vi "Set Crop ROI.vi"(8 "error in (no error)":errorcluster, 11 "Frame Grabber Data in":T2={"Camera Session"="", "Frame"=refnum, "AVI Refnum"=refnum, "Codecs"=[], "Frame number"=0, "Tracking File Refnum"=refnum, "Tick Count"=0, "Probe Object"=refnum, "Playback Probe Data"=[], "Rigid Body"={"Position"={"x (mm)"=0.0, "y (mm)"=0.0, "z (mm)"=0.0}, "Orientation"={"Pitch (rad)"=0.0, "Yaw (rad)"=0.0, "Roll (rad)"=0.0}, "Quaternion"={"qx"=0.0, "qy"=0.0, "qz"=0.0, "qw"=0.0}, "Tracked?"=FALSE}, "Total no frames playback"=0, "Video FPS"=0.0, "Camera connected?"=FALSE, "Scene"=refnum, "Cropped Frame"=refnum, "Tracker FPS"=0.0, "Crop ROI"=[], "Presentation Values"=[], "Elapsed time (ms)"=0, "Camera frames playback"=0, "Refnums"={"Live Refnum"=refnum, "Record Refnum"=refnum, "Recording Settings Refnum"=refnum, "Playback Refnum"=refnum, "Frame Slider Refnum"=refnum, "Pause Refnum"=refnum, "Home Refnum"=refnum, "Crop Refnum"=refnum, "Clear Crop Refnum"=refnum, "stop refnum"=refnum, "Playback Rate Refnum"=refnum, "Operator Settings Refnums"=refnum, "Presentation Refnum"=refnum, "Gestation Refnum"=refnum, "Connection Settings Refnum"=refnum, "Crop Time Frame Slider Refnum"=refnum, "Cancel Save Refnum"=refnum}, "Dimensions"={"Probe Dimensions"={"Probe Width"=0.0, "Probe Depth"=1.0, "Probe Height"=0.0}, "Room Dimensions"={"Room Width"=0.0, "Room Depth"=0.0, "Room Height"=0.0}}, "Playback Data As Strings"=[], "Cropped Tracking File Refnum"=refnum, "Cropped AVI Refnum"=refnum, "Header"=[]}) -> (0 "error out":errorcluster, 1 "Crop ROI":i32[](array[numeric]), 2 "Image Out":T1, 3 "Frame Grabber Data out":T2={"Camera Session"="", "Frame"=refnum, "AVI Refnum"=refnum, "Codecs"=[], "Frame number"=0, "Tracking File Refnum"=refnum, "Tick Count"=0, "Probe Object"=refnum, "Playback Probe Data"=[], "Rigid Body"={"Position"={"x (mm)"=0.0, "y (mm)"=0.0, "z (mm)"=0.0}, "Orientation"={"Pitch (rad)"=0.0, "Yaw (rad)"=0.0, "Roll (rad)"=0.0}, "Quaternion"={"qx"=0.0, "qy"=0.0, "qz"=0.0, "qw"=0.0}, "Tracked?"=FALSE}, "Total no frames playback"=0, "Video FPS"=0.0, "Camera connected?"=FALSE, "Scene"=refnum, "Cropped Frame"=refnum, "Tracker FPS"=0.0, "Crop ROI"=[], "Presentation Values"=[], "Elapsed time (ms)"=0, "Camera frames playback"=0, "Refnums"={"Live Refnum"=refnum, "Record Refnum"=refnum, "Recording Settings Refnum"=refnum, "Playback Refnum"=refnum, "Frame Slider Refnum"=refnum, "Pause Refnum"=refnum, "Home Refnum"=refnum, "Crop Refnum"=refnum, "Clear Crop Refnum"=refnum, "stop refnum"=refnum, "Playback Rate Refnum"=refnum, "Operator Settings Refnums"=refnum, "Presentation Refnum"=refnum, "Gestation Refnum"=refnum, "Connection Settings Refnum"=refnum, "Crop Time Frame Slider Refnum"=refnum, "Cancel Save Refnum"=refnum}, "Dimensions"={"Probe Dimensions"={"Probe Width"=0.0, "Probe Depth"=1.0, "Probe Height"=0.0}, "Room Dimensions"={"Room Width"=0.0, "Room Depth"=0.0, "Room Height"=0.0}}, "Playback Data As Strings"=[], "Cropped Tracking File Refnum"=refnum, "Cropped AVI Refnum"=refnum, "Header"=[]}, 5 "Zero crop size?":bool)   [LabVIEW 2017]
uses:
  Controls/Frame Grabber Data.ctl
  <vilib>/userdefined/High Color/IMAQdx.ctl
  <vilib>/vision/Image Controls.llb/IMAQ Image.ctl
  <vilib>/vision/Avi.llb/IMAQ AVI2 Refnum.ctl
  Controls/Rigid Body Info.ctl
  Controls/Position.ctl
  Controls/Orientation.ctl
  Controls/Refnums.ctl
  Controls/Recording Settings.ctl
  Controls/Operator Settings.ctl
  Controls/Operator.ctl
  Controls/Dimensions.ctl
  Controls/Room Dimensions.ctl
  <vilib>/vision/NI_Vision_Development_Module.lvlib
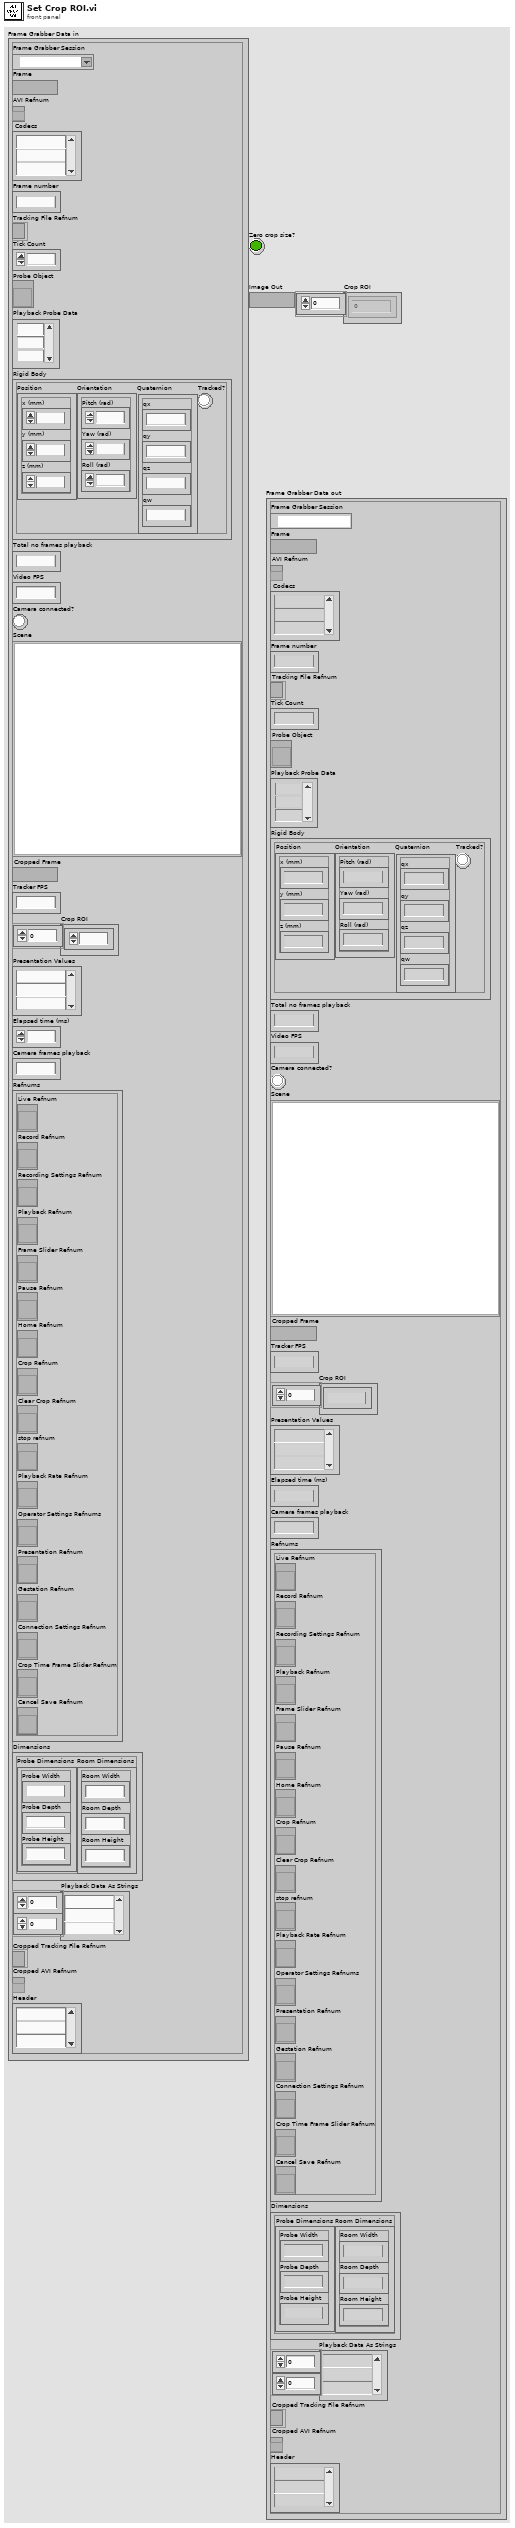
[diagram p1: front panel]
types:
  T1 = typedef "IMAQ Image.ctl" = refnum<image>
  T2 = typedef "Frame Grabber Data.ctl" = cluster{"Camera Session":T3, "Frame":T1, "AVI Refnum":T4, "Codecs":string[], "Frame number":u32, "Tracking File Refnum":refnum<file>, "Tick Count":u32, "Probe Object":refnum<vi>, "Playback Probe Data":dbl[][], "Rigid Body":T5, "Total no frames playback":i32, "Video FPS":dbl, "Camera connected?":bool, "Scene":refnum<vi>, "Cropped Frame":T1, "Tracker FPS":dbl, "Crop ROI":i32[], "Presentation Values":string[], "Elapsed time (ms)":u32, "Camera frames playback":u32, "Refnums":T8, "Dimensions":T9, "Playback Data As Strings":string[][], "Cropped Tracking File Refnum":refnum<file>, "Cropped AVI Refnum":T4, "Header":string[]}
  T3 = typedef "IMAQdx.ctl" = refnum<k21>
  T4 = typedef "IMAQ AVI2 Refnum.ctl" = refnum<k20>
  T5 = typedef "Rigid Body Info.ctl" = cluster{"Position":T6, "Orientation":T7, "Quaternion":cluster{"qx":sgl, "qy":sgl, "qz":sgl, "qw":sgl}, "Tracked?":bool}
  T6 = typedef "Position.ctl" = cluster{"x (mm)":sgl, "y (mm)":sgl, "z (mm)":sgl}
  T7 = typedef "Orientation.ctl" = cluster{"Pitch (rad)":sgl, "Yaw (rad)":sgl, "Roll (rad)":sgl}
  T8 = typedef "Refnums.ctl" = cluster{"Live Refnum":refnum<vi>, "Record Refnum":refnum<vi>, "Recording Settings Refnum":refnum<vi>, "Playback Refnum":refnum<vi>, "Frame Slider Refnum":refnum<vi>, "Pause Refnum":refnum<vi>, "Home Refnum":refnum<vi>, "Crop Refnum":refnum<vi>, "Clear Crop Refnum":refnum<vi>, "stop refnum":refnum<vi>, "Playback Rate Refnum":refnum<vi>, "Operator Settings Refnums":refnum<vi>, "Presentation Refnum":refnum<vi>, "Gestation Refnum":refnum<vi>, "Connection Settings Refnum":refnum<vi>, "Crop Time Frame Slider Refnum":refnum<vi>, "Cancel Save Refnum":refnum<vi>}
  T9 = typedef "Dimensions.ctl" = cluster{"Probe Dimensions":cluster{"Probe Width":sgl, "Probe Depth":sgl, "Probe Height":sgl}, "Room Dimensions":T10}
  T10 = typedef "Room Dimensions.ctl" = cluster{"Room Width":dbl, "Room Depth":dbl, "Room Height":dbl}
  T11 = typedef "IMAQ Rectangle" = cluster{"Left":i32, "Top":i32, "Right":i32, "Bottom":i32, "Rotation":dbl}
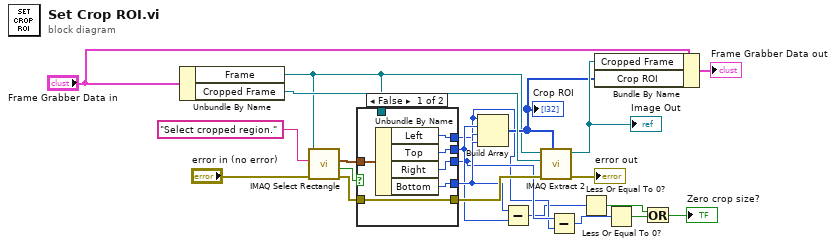
[diagram p0: block diagram]
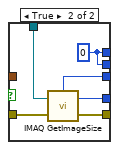
[diagram p2: hidden frame]
diagram:
  n1 = Unbundle By Name("Frame Grabber Data in") -> ("Frame"=w10:T1, "Cropped Frame"=w17:T1)
  n2 = call "IMAQ Select Rectangle"("error in (no error)"="error in (no error)", "Prompt"="Select cropped region.", "Image In"=w10) -> ("error out"=w12:errorcluster, "Cancelled"=w13:bool, "Rectangle"=w22:T11)  [unwired: 5 in, 1 out]
  n3 = case shown="False" w13 {
    tunnel: w22 -> [w28 _]
    tunnel: [w27 w32] -> w6
    tunnel: [w26 w32] -> w8
    tunnel: [w25 w30] -> w7
    tunnel: [w24 w31] -> w9
    tunnel: w12 -> [w23 w34]
    tunnel: [w23 w33] -> w11
    tunnel: w10 -> [_ w29]
    frame False {
      n4 = Unbundle By Name(w28) -> ("Left"=w27:i32, "Top"=w26:i32, "Right"=w25:i32, "Bottom"=w24:i32)
    }
    frame True {
      w32 = 0 ("Left")
      n5 = call "IMAQ GetImageSize"("Image"=w29, "error in (no error)"=w34) -> ("Y Resolution"=w31:i32, "X Resolution"=w30:i32, "error out"=w33:errorcluster)  [unwired: 2 in]
    }
  }
  n6 = Build Array(w6, w8, w7, w9) -> (w14:i32[])
  "Crop ROI" <- w14
  n7 = Subtract(x=w9, y=w8) -> (x-y=w4:i32)
  n8 = call "IMAQ Extract 2"("Optional Rectangle"=w14, "error in (no error)"=w11, "Image Dst"=w17, "Image Src"=w10) -> ("error out"=→"error out":errorcluster, "Image Dst Out"=w15:T1)  [unwired: 6 in]
  "Image Out" <- w15
  n9 = Subtract(x=w7, y=w6) -> (x-y=w5:i32)
  n10 = Less Or Equal To 0?(x=w4) -> (x <= 0?=w2:bool)
  n11 = Bundle By Name(cluster="Frame Grabber Data in", "Cropped Frame"=w15, "Crop ROI"=w14) -> (→"Frame Grabber Data out":T2)
  n12 = Less Or Equal To 0?(x=w5) -> (x <= 0?=w3:bool)
  n13 = Or(x=w2, y=w3) -> (x .or. y?=→"Zero crop size?":bool)
